vi "ClearNoise analisis.vi"(0 "summary temp A":u32[][](array[numeric]), 1 "summary temp B":u32[][](array[numeric]), 2 "Chip ID list 1":u16[](array[numeric]) format="%.0x", 3 "Chip ID list 2":u16[](array[numeric]) format="%.0x", 4 "Threshold Z":u32=1000) -> (5 "Killing list A":T1(array[cluster]) {"ChipID" format="%.0x"}, 6 "Killing list B":T1(array[cluster]) {"ChipID" format="%.0x"})   [LabVIEW 2015, in "VIPM2.lvlib"]
uses:
  VIPM2.lvlib
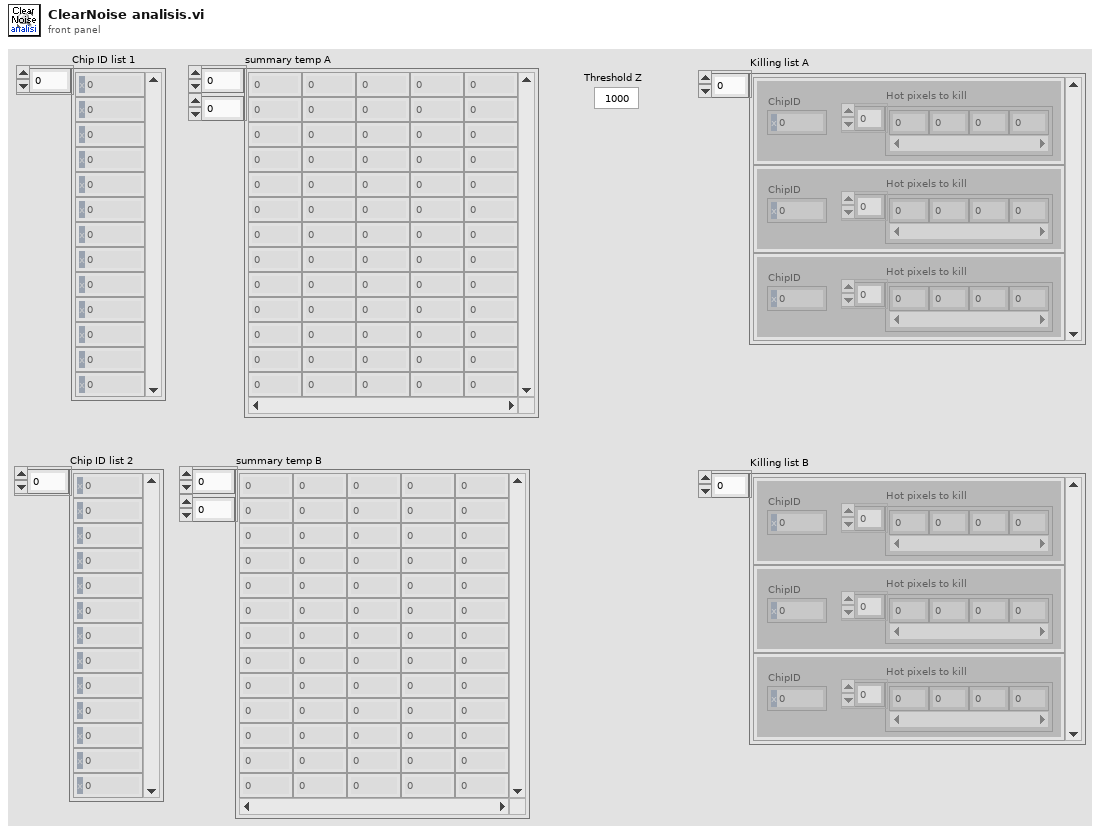
[diagram p1: front panel]
types:
  T1 = cluster{"ChipID":u16, "Hot pixels to kill":u8[]}[]
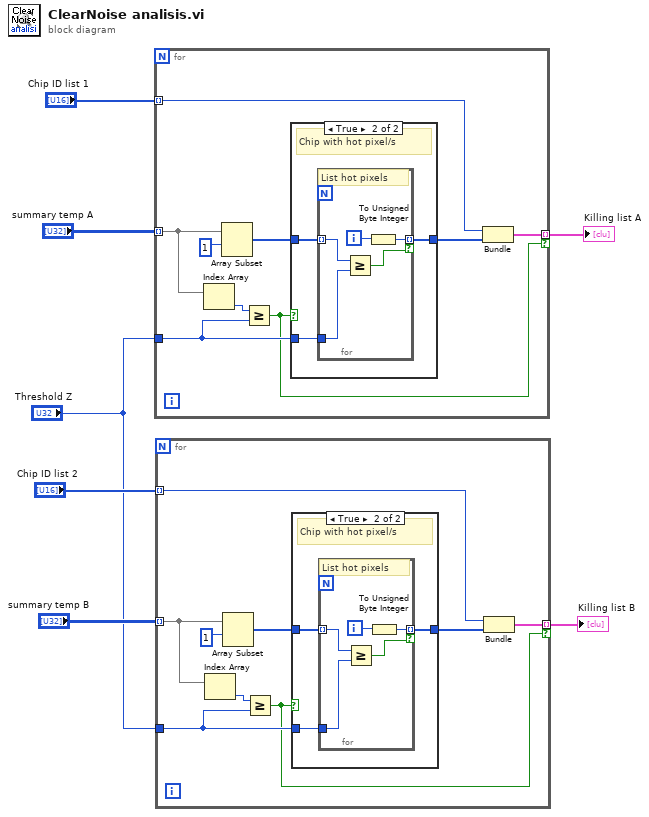
[diagram p0: block diagram]
diagram:
  n1 = for {
    tunnel: "Chip ID list 1" -> [w11] mode=indexing
    tunnel: "summary temp A" -> [w14] mode=indexing
    tunnel: "Threshold Z" -> [w15]
    tunnel: [w9] -> w5 mode=indexing if=w8
    n2 = Index Array "Index Array"(array=w14) -> (element=w16:u32)  [unwired: 1 in]
    n3 = Array Subset "Array Subset"(array=w14, index=1) -> (w12:u32[])  [unwired: 1 in]
    n4 = Greater Or Equal?(x=w16, y=w15) -> (x >= y?=w8:bool)
    n5 = case shown="True" w8 {
      tunnel: w15 -> [_ w19]
      tunnel: w12 -> [_ w18]
      tunnel: [_ w17] -> w10
      frame False {
        # "no hot pixels"
      }
      frame True {
        # "Chip with hot pixel/s"
        n6 = for {
          tunnel: w19 -> [w24]
          tunnel: w18 -> [w22] mode=indexing
          tunnel: [w21] -> w17 mode=indexing if=w23
          i -> [w20]
          # "List hot pixels"
          n7 = Greater Or Equal?(x=w22, y=w24) -> (x >= y?=w23:bool)
          n8 = To Unsigned Byte Integer(number=w20) -> (unsigned 8bit integer=w21:u8)
        }
      }
    }
    n9 = Bundle "Bundle"(w11, w10) -> (w9:cluster{u16, u8[]})  [unwired: 1 in]
  }
  "Killing list A" <- w5
  n10 = for {
    tunnel: "Chip ID list 2" -> [w28] mode=indexing
    tunnel: "summary temp B" -> [w31] mode=indexing
    tunnel: "Threshold Z" -> [w32]
    tunnel: [w26] -> w1 mode=indexing if=w25
    n11 = Index Array "Index Array"(array=w31) -> (element=w33:u32)  [unwired: 1 in]
    n12 = Array Subset "Array Subset"(array=w31, index=1) -> (w29:u32[])  [unwired: 1 in]
    n13 = Greater Or Equal?(x=w33, y=w32) -> (x >= y?=w25:bool)
    n14 = case shown="True" w25 {
      tunnel: w32 -> [_ w36]
      tunnel: w29 -> [_ w35]
      tunnel: [_ w34] -> w27
      frame False {
        # "no hot pixels"
      }
      frame True {
        # "Chip with hot pixel/s"
        n15 = for {
          tunnel: w36 -> [w41]
          tunnel: w35 -> [w39] mode=indexing
          tunnel: [w38] -> w34 mode=indexing if=w40
          i -> [w37]
          # "List hot pixels"
          n16 = Greater Or Equal?(x=w39, y=w41) -> (x >= y?=w40:bool)
          n17 = To Unsigned Byte Integer(number=w37) -> (unsigned 8bit integer=w38:u8)
        }
      }
    }
    n18 = Bundle "Bundle"(w28, w27) -> (w26:cluster{u16, u8[]})  [unwired: 1 in]
  }
  "Killing list B" <- w1
